vi "Pre-Process.vi"(11 "Arilou in":refnum<class "Slylandro.lvclass">) -> (3 "Arilou out":refnum<class "Slylandro.lvclass">)   [LabVIEW 2021, in "Slylandro.lvclass"]
uses:
  Slylandro.lvclass
  C:/dev/LabVIEW/LabMelee/Source/Application Specific/Ship/Ship.lvclass
  C:/dev/LabVIEW/LabMelee/Source/Application Specific/Element/Element.lvclass
  Ship/Ship.lvclass/Ship.ctl
  Control State/Control State.lvclass/Control State.ctl
  Slylandro.lvclass/Slylandro.ctl
  Element/Element.lvclass
  Control State/Control State.lvclass
  Ship/Ship.lvclass
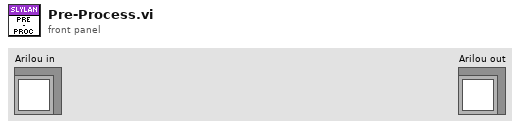
[diagram p1: front panel]
types:
  T1 = typedef "Control State.lvclass/Button State.ctl" = enum16{"Undefined", "Pressed", "Released", "Held", "Not Held"}
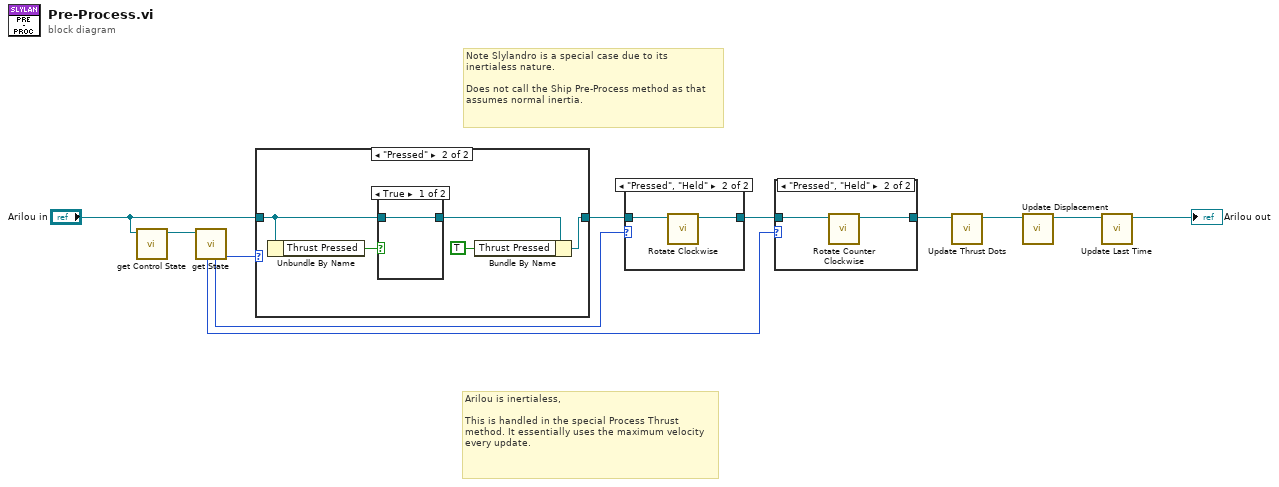
[diagram p0: block diagram]
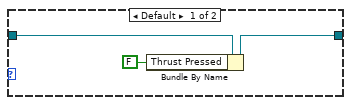
[diagram p4: hidden frame]
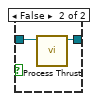
[diagram p5: hidden frame]
diagram:
  # "Note Slylandro is a special case due to its inertialess nature.\n\nDoes not call the Ship Pre-Process method as that assumes normal inertia."
  # "Arilou is inertialess, \n\nThis is handled in the special Process Thrust method. It essentially uses the maximum velocity every update."
  n1 = call "get Control State.vi"("Ship in"="Arilou in") -> ("Control State"=w2:refnum<class "Control State.lvclass">)  [unwired: 10 in]
  n2 = call "get State.vi"("Control State in"=w2) -> ("Thrust"=w9:T1, "Rotate Clockwise"=w8:T1, "Rotate Counter Clockwise"=w5:T1)  [unwired: 6 in, 2 out]
  n3 = case shown="\"Pressed\"" w9 {
    tunnel: "Arilou in" -> [w13 w16]
    tunnel: [w14 w18] -> w7
    frame Default {
      n4 = Bundle By Name(cluster=w13, "Thrust Pressed"=FALSE) -> (w14:refnum<class "Slylandro.lvclass">)
    }
    frame "Pressed" {
      n5 = Unbundle By Name(w16) -> ("Thrust Pressed"=w15:bool)
      n6 = case shown="True" w15 {
        tunnel: [w20 w22] -> w19
        tunnel: w16 -> [w20 w21]
        frame True {
        }
        frame False {
          n7 = call "Process Thrust.vi"("Arilou in"=w21) -> ("Arilou out"=w22:refnum<class "Slylandro.lvclass">)  [unwired: 10 in]
        }
      }
      n8 = Bundle By Name(cluster=w19, "Thrust Pressed"=TRUE) -> (w18:refnum<class "Slylandro.lvclass">)
    }
  }
  n9 = case shown="\"Pressed\", \"Held\"" w8 {
    tunnel: w7 -> [w23 w25]
    tunnel: [w23 w24] -> w6
    frame Default {
    }
    frame "Pressed", "Held" {
      n10 = call "Rotate Clockwise.vi"("Element in"=w25) -> ("Element out"=w24:refnum<class "Slylandro.lvclass">)  [unwired: 10 in]
    }
  }
  n11 = case shown="\"Pressed\", \"Held\"" w5 {
    tunnel: w6 -> [w26 w28]
    tunnel: [w26 w27] -> w10
    frame Default {
    }
    frame "Pressed", "Held" {
      n12 = call "Rotate Counter Clockwise.vi"("Element in"=w28) -> ("Element out"=w27:refnum<class "Slylandro.lvclass">)  [unwired: 10 in]
    }
  }
  n13 = call "Update Thrust Dots.vi"("Ship in"=w10) -> ("Ship out"=w4:refnum<class "Slylandro.lvclass">)  [unwired: 10 in]
  n14 = call "Update Displacement.vi"("Element in"=w4) -> ("Element out"=w11:refnum<class "Slylandro.lvclass">)  [unwired: 10 in]
  n15 = call "Update Last Time.vi"("Element in"=w11) -> ("Element out"=→"Arilou out":refnum<class "Slylandro.lvclass">)  [unwired: 10 in]
